vi "AddOperationRun.vi"(6 "OperationStatus (NOT_COMPLETED)":T1=enum."NOT_COMPLETED", 7 "OperationRunStartTime (Now)":timestamp, 8 "error in":errorcluster, 10 "OperationName (Generic_Operation)":string="Generic_Operation", 11 "ProcessRun in":refnum<class "ProcessRun.lvclass">) -> (0 "error out":errorcluster, 2 "OperationRun":refnum<class "OperationRun.lvclass">, 3 "ProcessRun out":refnum<class "ProcessRun.lvclass">)   [LabVIEW 2021, in "ProligentXMLGenerator.lvlib" / "ProcessRun.lvclass"]
doc: "Add an OperationRun.\n\nDefines the operation run, a logical container for the execution of sequences and processes.\nOperation runs are globaly unique by their OperationRunId property."
uses:
  ProcessRun.lvclass
  ProcessRun.lvclass/ProcessRun.ctl
  OperationRun/OperationRun.lvclass
  Base/ExecutionStatus/Value.ctl
  Base/ExecutionStatus/ExecutionStatus.lvclass
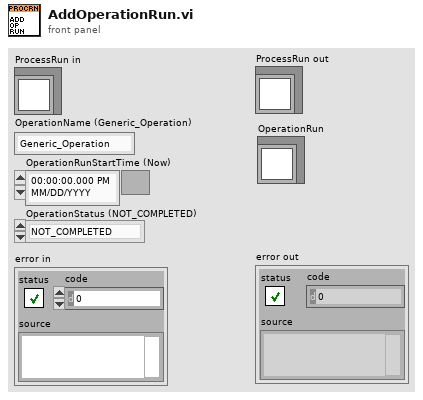
[diagram p1: front panel]
types:
  T1 = typedef "ProligentXMLGenerator.lvlib/ExecutionStatus.lvclass/Value.ctl" = enum16{"PASS", "FAIL", "NOT_COMPLETED", "ABORTED"}
  T2 = typedef "ProligentXMLGenerator.lvlib/ProcessRun.lvclass/Data.ctl" = cluster{"Name":string, "OperationRuns":refnum<class "OperationRun.lvclass">[], "OperationCycles":refnum<class "OperationCycle.lvclass">[], "FailureReferences":refnum<class "FailureReference.lvclass">[], "CustomData":refnum<class "CustomData.lvclass">, "ProcessRunId":refnum<class "Guid.lvclass">, "ProcessFullName":refnum<class "ProcessFullName.lvclass">, "ProcessVersion":refnum<class "NonEmptyString_64.lvclass">, "ProductUnitIdentifier":refnum<class "NonEmptyString_50.lvclass">, "ProductFullName":refnum<class "FullName.lvclass">, "ProcessRunStatus":refnum<class "ExecutionStatus.lvclass">, "ProcessRunStartTime":refnum<class "DateTime.lvclass">, "ProcessRunEndTime":refnum<class "DateTime.lvclass">, "ProcessMode":refnum<class "NonEmptyString_64.lvclass">, "TimeZoneInfoId":string}
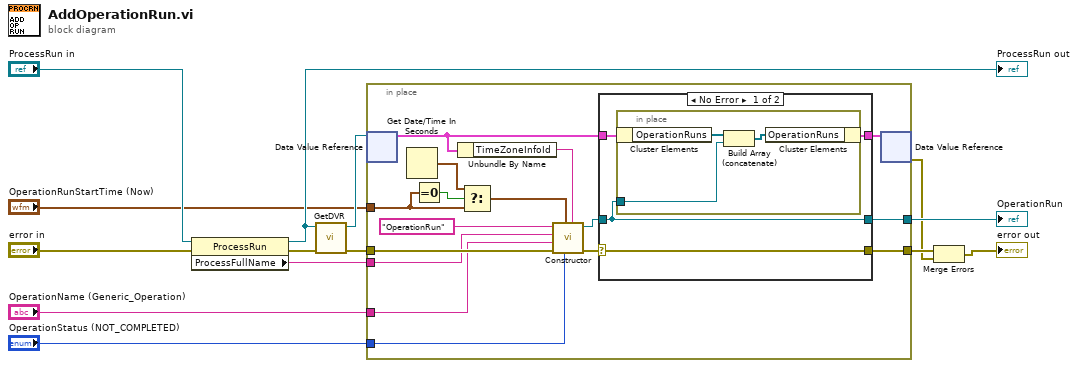
[diagram p0: block diagram]
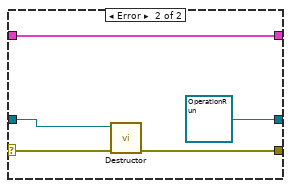
[diagram p2: hidden frame]
diagram:
  n1 = property on="Property Node" class="ProcessRun"(reference="ProcessRun in", error in="error in") -> (reference out=w3:refnum<class "ProcessRun.lvclass">, error out=w5:errorcluster, "ProcessFullName"=w2:string)
  "ProcessRun out" <- w3
  n2 = call "GetDVR.vi"("error in"=w5, "ProcessRun"=w3) -> ("error out"=w8:errorcluster, "DVRReference"=w7:refnum<data-value>)  [unwired: 8 in]
  n3 = in-place "In Place Element Structure" {
    in-place-border: [w29] -> w9
    in-place-border: w8 -> [w28]
    in-place-border: [w26] -> w12
    in-place-border: "OperationStatus (NOT_COMPLETED)" -> [w22]
    in-place-border: "OperationName (Generic_Operation)" -> [w23]
    in-place-border: w2 -> [w21]
    in-place-border: "OperationRunStartTime (Now)" -> [w18]
    n4 = in-place-dvr #1(w7) -> (w16:T2)  [unwired: 1 out]
    n5 = Get Date/Time In Seconds() -> (seconds since 1Jan1904=w19:timestamp)
    n6 = Equal To 0?(x=w18) -> (x = 0?=w20:bool)
    n7 = Unbundle By Name(w16) -> ("TimeZoneInfoId"=w15:string)
    n8 = Select(t=w19, s=w20, f=w18) -> (s? t:f=w17:timestamp)
    n9 = call "Constructor.vi"("TimeZoneInfoId"=w15, "OperationStatus"=w22, "OperationRunStartTime"=w17, "error in"=w28, "OperationName"=w23, "ProcessFullName"=w21, "Name"="OperationRun") -> ("error out"=w30:errorcluster, "OperationRun out"=w25:refnum<class "OperationRun.lvclass">)  [unwired: 3 in]
    n10 = case shown="No Error" w30 {
      selector: w30 -> [w34 w41]
      tunnel: [w31 w42] -> w27
      tunnel: [w34 w40] -> w29
      tunnel: w25 -> [w33 w39]
      tunnel: w16 -> [w32 w42]
      tunnel: [w33 refnum<class "OperationRun.lvclass"> refnum ("ProligentResultProcessor:OperationRun")] -> w26
      frame No Error {
        n11 = in-place "In Place Element Structure" {
          in-place-border: w33 -> [w37]
          n12 = in-place-cluster #2(w32) -> ("OperationRuns"=w36:refnum<class "OperationRun.lvclass">[])
          n13 = Build Array (concatenate)(w36, w37) -> (w35:refnum<class "OperationRun.lvclass">[])
          n14 = in-place-cluster #2("OperationRuns"=w35) -> (w31:T2)
        }
      }
      frame Error {
        n15 = call "Destructor.vi"("error in"=w41, "OperationRun"=w39) -> ("error out"=w40:errorcluster)  [unwired: 9 in]
      }
    }
    n16 = in-place-dvr #1(w27) -> (w6:errorcluster)  [unwired: 1 out]
  }
  "OperationRun" <- w12
  n17 = Merge Errors(w9, w6) -> (→"error out":errorcluster)
